vi "Write Latest movie role.vi"(8 "error in (no error)":errorcluster, 10 "Latest movie role":string, 11 "John Cena in":refnum<class "John Cena.lvclass">) -> (0 "error out":errorcluster, 3 "John Cena out":refnum<class "John Cena.lvclass">)   [LabVIEW 2019, in "John Cena.lvclass"]
uses:
  John Cena.lvclass
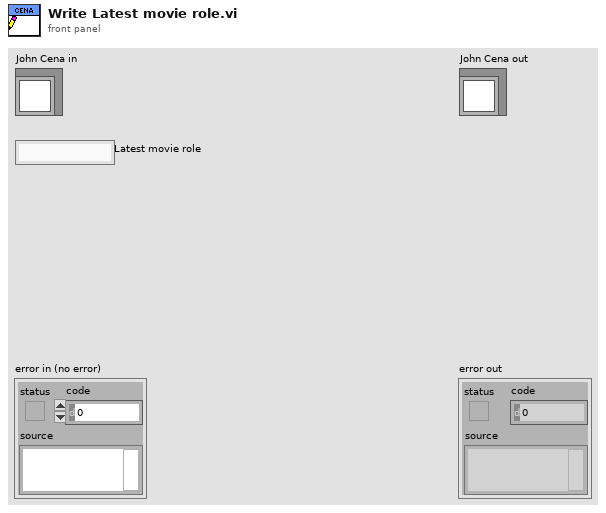
[diagram p1: front panel]
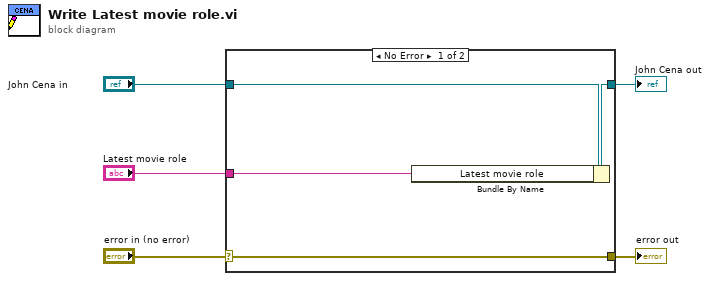
[diagram p0: block diagram]
diagram:
  n1 = case shown="No Error" "error in (no error)" {
    selector: "error in (no error)" -> [w9 w10]
    tunnel: [w9 w10] -> w4
    tunnel: [w7 w11] -> w2
    tunnel: "John Cena in" -> [w8 w11]
    tunnel: "Latest movie role" -> [w6 _]
    frame No Error {
      n2 = Bundle By Name(cluster=w8, "Latest movie role"=w6) -> (w7:refnum<class "John Cena.lvclass">)
    }
    frame Error {
    }
  }
  "error out" <- w4
  "John Cena out" <- w2
